vi "Absolute Value (Components).vi"(11 "A":refnum<class "Vector 2D.lvclass">) -> (3 "Absolute A":refnum<class "Vector 2D.lvclass">)   [LabVIEW 2021, in "Vector 2D.lvclass"]
uses:
  Vector 2D.lvclass
  Vector 2D.lvclass/Vector 2D.ctl
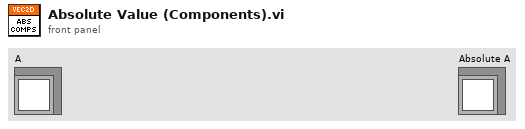
[diagram p1: front panel]
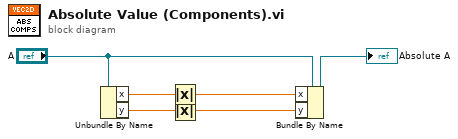
[diagram p0: block diagram]
diagram:
  n1 = Unbundle By Name("A") -> ("x"=w4:sgl, "y"=w2:sgl)
  n2 = Absolute Value(x=w4) -> (abs(x)=w3:sgl)
  n3 = Absolute Value(x=w2) -> (abs(x)=w1:sgl)
  n4 = Bundle By Name(cluster="A", "x"=w3, "y"=w1) -> (→"Absolute A":refnum<class "Vector 2D.lvclass">)
